vi "DSF Data Viewer.vi"(6 "menu options":cluster{"open":bool, "save":bool, "view":bool}={"open"=TRUE, "save"=FALSE, "view"=FALSE}, 8 "error in (no error)":errorcluster, 9 "Stop Pointer":refnum<class "Pointer.lvclass">, 10 "Framework Configuration":T1, 11 "DSF":refnum<class "Framework.lvclass">) -> (0 "error out":errorcluster)   [LabVIEW 2017, in "DSF Data Viewer.lvlib"]
uses:
  DSF Data Viewer.lvlib
  Builds/Data Sharing Framework/Current/Core/DSF Core.lvlibp/Engine/Classes/Framework/Framework.lvclass
  Builds/Data Sharing Framework/Current/Core/DSF Core.lvlibp/DSF Configuration API/Public/Controls/DSF Engine Framework Configuration.ctl
  Builds/Data Sharing Framework/Current/Core/DSF Core.lvlibp/DSF Configuration API/Public/Controls/DSF Engine Plugin Configuration.ctl
  Builds/Data Sharing Framework/Current/Core/DSF Core.lvlibp/DSF Configuration API/Public/Controls/DSF Timing Info.ctl
  Builds/Data Sharing Framework/Current/Core/DSF Core.lvlibp/DSF Configuration API/Public/Controls/DSF Engine Plugin Thread Configuration.ctl
  Builds/Data Sharing Framework/Current/Core/DSF Core.lvlibp/DSF Configuration API/Public/Controls/DSF Settings Info.ctl
  Builds/Data Sharing Framework/Current/Core/DSF Core.lvlibp/DSF Configuration API/Public/Controls/DSF Engine Transfer Group Configuration.ctl
  Builds/Data Sharing Framework/Current/Core/DSF Core.lvlibp/DSF Configuration API/Public/Controls/DSF Direction.ctl
  Builds/Data Sharing Framework/Current/Core/DSF Core.lvlibp/DSF Configuration API/Public/Controls/DSF Engine Transfer Configuration.ctl
  Builds/Data Sharing Framework/Current/Core/DSF Core.lvlibp/DSF Configuration API/Public/Controls/DSF Byte Order.ctl
  Builds/Data Sharing Framework/Current/Core/DSF Core.lvlibp/DSF Configuration API/Public/Controls/DSF Engine Channel Configuration.ctl
  Builds/Data Sharing Framework/Current/Core/DSF Core.lvlibp/DSF Configuration API/Public/Controls/DSF Data Type.ctl
  <vilib>/NI/Memory Manager/Classes/Pointer/Pointer.lvclass
  Source/Main VI/Application Data.ctl
  Source/Buffer Reader/Buffer Data.ctl
  Builds/Data Sharing Framework/Current/Core/DSF Core.lvlibp/Engine/Classes/Buffer/Buffer.lvclass
  <vilib>/NI/Memory Manager/Classes/Pointer/Pointer.lvclass/Pointer.ctl
  <vilib>/NI/Memory Manager/Classes/Pointer/Write Bool.vi
  <vilib>/NI/Memory Manager/Classes/Pointer/Read Bool.vi
  <vilib>/NI/Memory Manager/Classes/Pointer/Get Address.vi
  <vilib>/NI/Memory Manager/Classes/Pointer/Write (No Check).vi
  <vilib>/NI/Memory Manager/Classes/Pointer/Write (No Check) Bool.vi
  <vilib>/NI/Memory Manager/Classes/Pointer/Check Move.vi
  <vilib>/NI/Memory Manager/Classes/Pointer/Read (No Check).vi
  <vilib>/NI/Memory Manager/Classes/Pointer/Read (No Check) Bool.vi
  <vilib>/NI/Memory Manager/Classes/Pointer/Check Null Pointer.vi
  <vilib>/NI/Memory Manager/Classes/Pointer/Check Count.vi
  <vilib>/NI/Memory Manager/Classes/Pointer/Check Bounds (Power of 2).vi
  <vilib>/NI/Memory Manager/Classes/Pointer/Errors.vi
  <vilib>/NI/Memory Manager/Classes/Pointer/Null Pointer.vi
  <vilib>/NI/Memory Manager/Classes/Pointer/Get Size.vi
  <vilib>/NI/Memory Manager/Classes/Pointer/Out of Bounds.vi
  <vilib>/NI/Memory Manager/Classes/Pointer/Check Bounds.vi
  <vilib>/NI/Memory Manager/Classes/Pointer/Create Error.vi
  <vilib>/NI/Memory Manager/VIs/Source.Write.String.vi
  <vilib>/NI/Memory Manager/Classes/Pointer/Write Pointer Size.vi
  <vilib>/NI/Memory Manager/VIs/Source.Write.Scalar.Base10.vi
  <vilib>/NI/Memory Manager/VIs/Source.Write.Scalar.Base10 (U64).vi
  <vilib>/NI/Memory Manager/Classes/Pointer/Check Pointer Bounds.vi
  <vilib>/NI/Memory Manager/Classes/Pointer/Check Buffer Bounds.vi
  <vilib>/NI/Memory Manager/VIs/New Error Cluster Constant.vi
  <vilib>/NI/Memory Manager/VIs/New Error Cluster Constant (512B).vi
  <vilib>/NI/Memory Manager/VIs/Error Cluster.Set Status.vi
  <vilib>/NI/Memory Manager/VIs/Error Cluster.Set Code.vi
  <vilib>/NI/Memory Manager/VIs/Error Cluster.Set VI Source.vi
  <vilib>/NI/Memory Manager/Constants/Constants.vi
  <vilib>/NI/Memory Manager/Constants/Library Name.vi
  <vilib>/NI/Memory Manager/Classes/Pointer/Pointer Error Info.vi
  <vilib>/NI/Memory Manager/Constants/Pointer Class Name.vi
  <vilib>/NI/Memory Manager/Classes/Pointer/Buffer Underflow.vi
  Builds/Data Sharing Framework/Current/Core/DSF Core.lvlibp/DSF Configuration API/Public/Largest Buffer Size (Framework).vi
  Builds/Data Sharing Framework/Current/Core/DSF Core.lvlibp/Engine/Classes/Buffer/Read Buffer String.vi
  Builds/Data Sharing Framework/Current/Core/DSF Core.lvlibp
  Builds/Data Sharing Framework/Current/Core/DSF Core.lvlibp/Engine/Classes/Status/Framework Performance.lvclass
panel:
  in  "Item Tree":string(tree)
  out "Frequency":dbl format="%.1fHz"
  out "Size":u64 format="%#_3pB"
  out "Null":bool
  out "Decimation":u64
  out "Throughput":dbl format="%.0pB/s"
  out "Buffer":string
  # "Data Viewer"
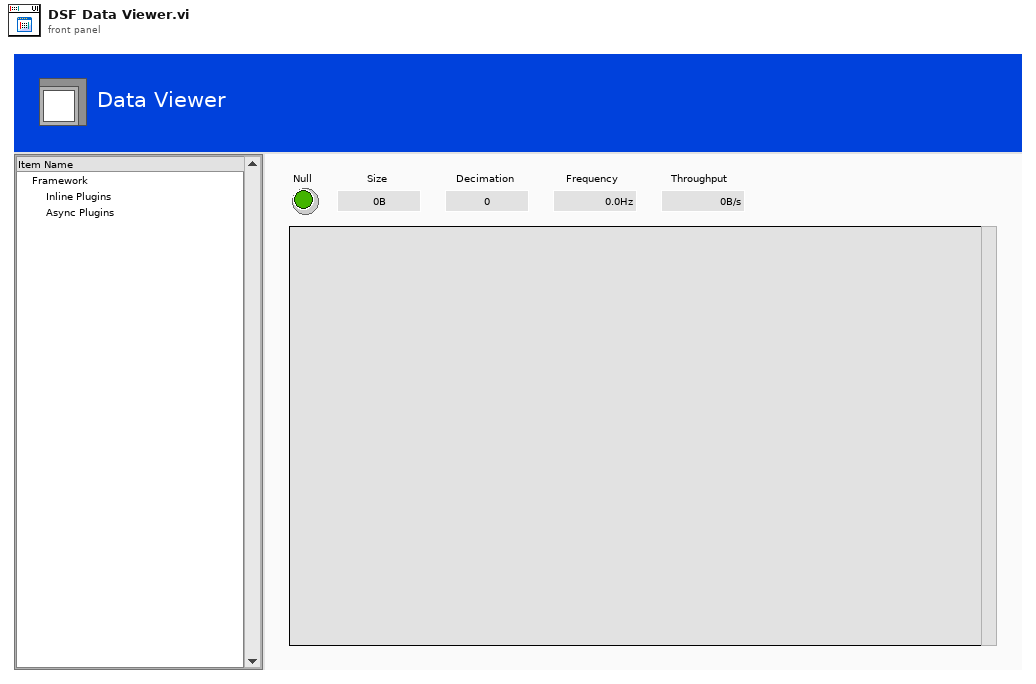
[diagram p1: front panel]
types:
  T1 = typedef "DSF Core.lvlibp/DSF Engine Framework Configuration.ctl" = cluster{"components directory":path, "Plugins":T2[]}
  T2 = typedef "DSF Core.lvlibp/DSF Engine Plugin Configuration.ctl" = cluster{"name":string, "components":string[], "cycle timing":T3, "threads":T4[], "Transfer Groups":T6[], "settings":T5}
  T3 = typedef "DSF Core.lvlibp/DSF Timing Info.ctl" = cluster{"priority":u64, "decimation":u64, "offset":u64}
  T4 = typedef "DSF Core.lvlibp/DSF Engine Plugin Thread Configuration.ctl" = cluster{"buffer converter settings":T5, "transceiver settings":T5, "processor":i32}
  T5 = typedef "DSF Core.lvlibp/DSF Settings Info.ctl" = cluster{"key":string, "value":string}[]
  T6 = typedef "DSF Core.lvlibp/DSF Engine Transfer Group Configuration.ctl" = cluster{"name":string, "direction":T7, "cycle timing":T3, "thread":i32, "settings":T5, "Transfers":T8[]}
  T7 = typedef "DSF Core.lvlibp/DSF Direction.ctl" = enum8{"Tx", "Rx"}
  T8 = typedef "DSF Core.lvlibp/DSF Engine Transfer Configuration.ctl" = cluster{"name":string, "byte order":T9, "settings":T5, "channels":T10[]}
  T9 = typedef "DSF Core.lvlibp/DSF Byte Order.ctl" = enum8{"big-endian", "little-endian"}
  T10 = typedef "DSF Core.lvlibp/DSF Engine Channel Configuration.ctl" = cluster{"string offset":u64, "string data type":T11, "engine data type":T11, "name":string, "settings":T5}
  T11 = typedef "DSF Core.lvlibp/DSF Data Type.ctl" = enum8{"Bool", "SGL", "DBL", "I8", "I16", "I32", "I64", "U8", "U16", "U32", "U64"}
  T12 = typedef "DSF Data Viewer.lvlib/Buffer Data.ctl" = cluster{"Buffer":refnum<class "Buffer.lvclass">, "decimation":u64}
  T13 = typedef "DSF Data Viewer.lvlib/Application Data.ctl" = cluster{"Item Tree Control":refnum<vi>, "Top-Level VI":refnum<vi>, "menu reference":refnum<k9>, "DSF":refnum<class "Framework.lvclass">, "buffer queue":refnum<queue>, "Stop Pointer":refnum<class "Pointer.lvclass">, "Buffer Variant":variant}
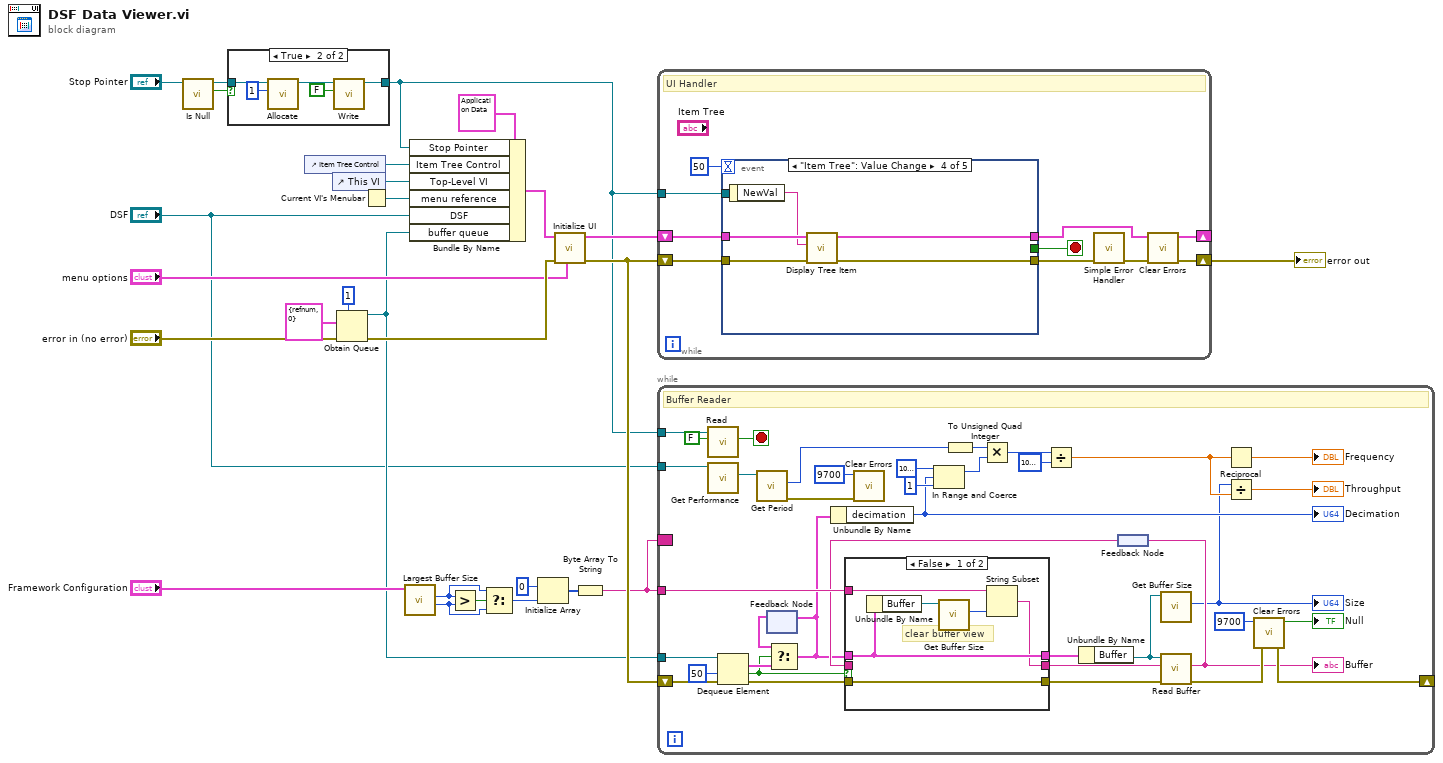
[diagram p0: block diagram]
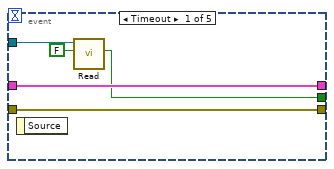
[diagram p4: hidden frame]
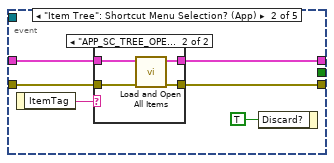
[diagram p5: hidden frame]
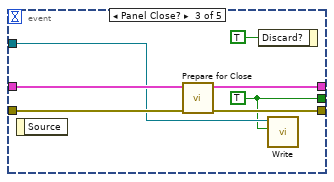
[diagram p7: hidden frame]
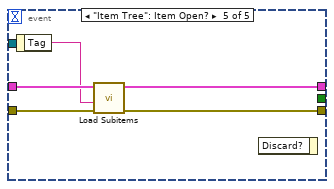
[diagram p8: hidden frame]
diagram:
  n1 = call <vilib>:"Is Null.vi"("Pointer in"="Stop Pointer") -> ("null?"=w6:bool)  [unwired: 8 in, 2 out]
  n2 = case shown="True" w6 {
    tunnel: [w27 w29] -> w4
    tunnel: "Stop Pointer" -> [w27 w31]
    frame False {
    }
    frame True {
      n3 = call-dynamic "Allocate.vi"("size"=u64 1, "Pointer in"=w31) -> ("Pointer out"=w30:refnum<class "Pointer.lvclass">)  [unwired: 8 in, 1 out]
      n4 = call-poly <vilib>:"Write.vi"("buffer in"=FALSE, "Pointer in"=w30) -> ("Pointer out"=w29:refnum<class "Pointer.lvclass">)  [unwired: 6 in, 3 out]
    }
  }
  n5 = control-ref of="Item Tree Control"() -> (w22:refnum<vi>)
  n6 = control-ref of="This VI"() -> (w25:refnum<vi>)
  n7 = Obtain Queue(max queue size (-1, unlimited)=1, element data type=T12 {"Buffer"=refnum, "decimation"=0} ("Buffer data"), error in (no error)="error in (no error)") -> (queue out=w3:refnum<queue>, error out=w18:errorcluster)  [unwired: 2 in, 1 out]
  n8 = Current VI's Menubar() -> (w23:refnum<k9>)
  n9 = call-poly "Largest Buffer Size.vi"("Framework Configuration in"="Framework Configuration") -> ("largest engine buffer size"=w14:u64, "largest string buffer size"=w15:u64)  [unwired: 7 in, 2 out]
  n10 = Bundle By Name(cluster=T13 {"Item Tree Control"=refnum, "Top-Level VI"=refnum, "menu reference"=refnum, "DSF"=refnum, "buffer queue"=refnum, "Stop Pointer"=refnum, "Buffer Variant"=variant}, "Stop Pointer"=w4, "Item Tree Control"=w22, "Top-Level VI"=w25, "menu reference"=w23, "DSF"="DSF", "buffer queue"=w3) -> (w21:T13)
  n11 = Greater?(x=w15, y=w14) -> (0:w16:bool)
  n12 = Select(t=w15, s=w16, f=w14) -> (s? t:f=w12:u64)
  n13 = Initialize Array(u8 0 ("element"), w12) -> (w11:u8[])
  n14 = call "Initialize UI.vi"("menu options"="menu options", "error in (no error)"=w18, "Application Data in"=w21) -> ("error out"=w5:errorcluster, "Application Data out"=w9:T13)  [unwired: 7 in]
  n15 = Byte Array To String(unsigned byte array=w11) -> (string=w2:string)
  n16 = while {
    shift-right: [w37] -> w24
    shift-left: w5 -> [w41]
    shift-right: [w38] -> _
    shift-left: w9 -> [w36]
    tunnel: w4 -> [w34]
    stop <- w35 stop-if-true
    # "UI Handler"
    n17 = event shown="[3] \"Item Tree\": Value Change" {
      selector: _ -> [_ _ _ _ _]
      dyn-events: _ -> [_ _ _ _ _]
      timeout: 50 -> [_ _ _ _ _]
      tunnel: [w42 _ w59 _ _] -> w35
      tunnel: w41 -> [w46 w49 w65 w70 w75]
      tunnel: [w46 w50 w63 w69 w74] -> w39
      tunnel: w36 -> [w45 w51 w61 w67 w73]
      tunnel: [w45 w47 w62 w68 w72] -> w38
      tunnel: w34 -> [w44 _ w60 _ _]
      event Timeout {
        n18 = event-data() -> ()  [unwired: 1 in, 1 out]
        n19 = call-poly <vilib>:"Read.vi"("buffer in"=FALSE, "Pointer in"=w44) -> ("buffer out"=w42:bool)  [unwired: 6 in, 3 out]
      }
      event "Item Tree": Shortcut Menu Selection? (App) {
        n20 = event-data() -> ("ItemTag"=w52:string)  [unwired: 1 in]
        n21 = case shown="\"APP_SC_TREE_OPEN_ALL_ITEMS\"" w52 {
          tunnel: w51 -> [w53 w58]
          tunnel: [w54 w56] -> w50
          tunnel: w49 -> [w54 w57]
          tunnel: [w53 w55] -> w47
          frame Default {
          }
          frame "APP_SC_TREE_OPEN_ALL_ITEMS" {
            n22 = call "Load and Open All Items.vi"("error in (no error)"=w57, "Application Data in"=w58) -> ("error out"=w56:errorcluster, "Application Data out"=w55:T13)  [unwired: 8 in]
          }
        }
        n23 = event-data("Discard?"=TRUE) -> ()  [unwired: 1 in, 1 out]
      }
      event Panel Close? {
        w59 = TRUE
        n24 = event-data() -> ()  [unwired: 1 in, 1 out]
        n25 = call "Prepare for Close.vi"("error in (no error)"=w65, "Application Data in"=w61) -> ("error out"=w63:errorcluster, "Application Data out"=w62:T13)  [unwired: 8 in]
        n26 = event-data("Discard?"=TRUE) -> ()  [unwired: 1 in, 1 out]
        n27 = call-poly <vilib>:"Write.vi"("buffer in"=w59, "Pointer in"=w60) -> ()  [unwired: 6 in, 4 out]
      }
      event "Item Tree": Value Change {
        n28 = event-data() -> ("NewVal"=w66:string)  [unwired: 1 in]
        n29 = call "Display Tree Item.vi"("error in (no error)"=w70, "Tag"=w66, "Application Data in"=w67) -> ("error out"=w69:errorcluster, "Application Data out"=w68:T13)  [unwired: 7 in]
      }
      event "Item Tree": Item Open? {
        n30 = event-data() -> ("Tag"=w71:string)  [unwired: 1 in]
        n31 = call "Load Subitems.vi"("error in (no error)"=w75, "Tag"=w71, "Application Data in"=w73) -> ("error out"=w74:errorcluster, "Application Data out"=w72:T13)  [unwired: 6 in, 1 out]
        n32 = event-data() -> ()  [unwired: 2 in, 1 out]
      }
    }
    n33 = call <vilib>:"Simple Error Handler.vi"("error in (no error)"=w39) -> ("error out"=w40:errorcluster)  [unwired: 4 in, 4 out]
    n34 = call <vilib>:"Clear Errors.vi"("error in (no error)"=w40) -> ("error out"=w37:errorcluster)  [unwired: 5 in, 1 out]
  }
  "error out" <- w24
  n35 = while {
    tunnel: w3 -> [w112]
    shift-right: [w83] -> _
    shift-left: w5 -> [w109]
    tunnel: w2 -> [w99]
    tunnel: w4 -> [w103]
    tunnel: "DSF" -> [w93]
    border: w2 -> [_]
    stop <- w104 stop-if-true
    # "Buffer Reader"
    n36 = call-poly <vilib>:"Read.vi"("buffer in"=FALSE, "Pointer in"=w103) -> ("buffer out"=w104:bool)  [unwired: 6 in, 3 out]
    n37 = call "Get Performance.vi"("Framework in"=w93) -> ("Performance"=w92:refnum<class "Framework Performance.lvclass">)  [unwired: 9 in, 1 out]
    n38 = Dequeue Element(queue=w112, timeout in ms (-1)=50, error in (no error)=w109) -> (element=w110:T12, timed out?=w100:bool, error out=w113:errorcluster)  [unwired: 1 out]
    n39 = call "Get Period.vi"("Framework Performance in"=w92) -> ("error out"=w76:errorcluster, "period"=w90:u32)  [unwired: 8 in, 1 out]
    n40 = feedback #1() -> (w98:T12)  [unwired: 1 in]
    n41 = Select(t=w98, s=w100, f=w110) -> (s? t:f=w80:T12)
    n42 = feedback-in #1(w80) -> ()
    n43 = Unbundle By Name(w80) -> ("decimation"=w86:u64)
    "Decimation" <- w86
    n44 = call <vilib>:"Clear Errors.vi"("error in (no error)"=w76, "specific error code to clear (0: all)"=9700) -> ()  [unwired: 4 in, 2 out]
    n45 = In Range and Coerce(upper limit=u64 1000000000, x=w86, lower limit=u64 1) -> (coerced(x)=w87:u64)  [unwired: 1 out]
    n46 = To Unsigned Quad Integer(1:w90) -> (0:w89:u64)
    n47 = Multiply(x=w89, y=w87) -> (x*y=w108:u64)
    n48 = Divide(x=w108, y=u64 1000000) -> (x/y=w88:dbl)
    n49 = feedback #2() -> (w96:string)
    n50 = case shown="False" w100 {
      tunnel: w96 -> [_ w122]
      tunnel: w80 -> [w115 w121]
      tunnel: w99 -> [w119 _]
      tunnel: [w114 w122] -> w94
      tunnel: w113 -> [w116 w120]
      tunnel: [w115 w121] -> w91
      tunnel: [w116 w120] -> w95
      frame False {
        # "clear buffer view"
        n51 = Unbundle By Name(w115) -> ("Buffer"=w117:refnum<class "Buffer.lvclass">)
        n52 = call "Get Buffer Size.vi"("Buffer in"=w117) -> ("buffer size"=w118:u64)  [unwired: 9 in, 1 out]
        n53 = String Subset(string=w119, length (rest)=w118) -> (substring=w114:string)  [unwired: 1 in]
      }
      frame True {
      }
    }
    n54 = Unbundle By Name(w91) -> ("Buffer"=w85:refnum<class "Buffer.lvclass">)
    n55 = call "Get Buffer Size.vi"("Buffer in"=w85) -> ("buffer size"=w78:u64)  [unwired: 9 in, 1 out]
    "Size" <- w78
    n56 = call-poly "Read Buffer.vi"("error in (no error)"=w95, "dst string in"=w94, "Buffer in"=w85) -> ("error out"=w84:errorcluster, "dst string out"=w79:string)  [unwired: 5 in, 2 out]
    "Buffer" <- w79
    n57 = feedback-in #2(w79) -> ()
    n58 = Reciprocal(x=w88) -> (1/x=→"Frequency":dbl)
    n59 = Divide(x=w78, y=w88) -> (x/y=→"Throughput":dbl)
    n60 = call <vilib>:"Clear Errors.vi"("error in (no error)"=w84, "specific error code to clear (0: all)"=9700) -> ("error out"=w83:errorcluster, "specific error cleared?"=→"Null":bool)  [unwired: 4 in]
  }
